vi "Log_Disdrometer_Raw_String.vi"(10 "FileFolder":path, 11 "Response":string) -> (0 "error out":errorcluster)   [LabVIEW 2018]
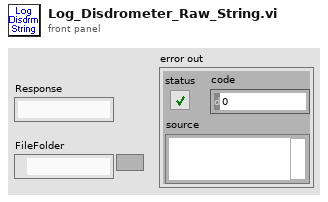
[diagram p1: front panel]
types:
  T1 = enum16{"open", "replace", "create", "open or create", "replace or create", "replace or create with confirmation"}
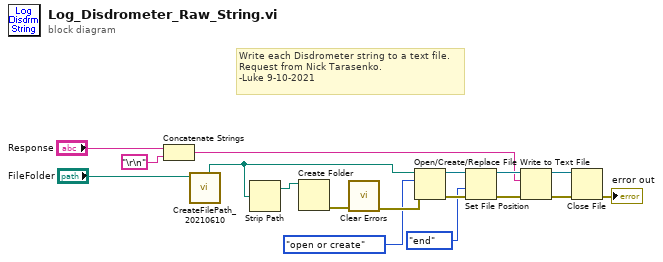
[diagram p0: block diagram]
diagram:
  # "Write each Disdrometer string to a text file.\nRequest from Nick Tarasenko. \n-Luke 9-10-2021"
  n1 = Concatenate Strings("Response", "\r\n") -> (w5:string)
  n2 = call "CreateFilePath_20210610.vi"("base path"="FileFolder") -> ("Disdrom_Raw_String_File"=w17:path)  [unwired: 6 in, 4 out]
  n3 = Strip Path(path=w17) -> (stripped path=w7:path)  [unwired: 1 out]
  n4 = Create Folder(path (use dialog)=w7) -> (error out=w8:errorcluster)  [unwired: 2 in, 2 out]
  n5 = call <vilib>:"Clear Errors.vi"("error in (no error)"=w8) -> ("error out"=w16:errorcluster)  [unwired: 5 in, 1 out]
  n6 = Open/Create/Replace File(file path (use dialog)=w17, error in=w16, operation (0:open)=T1."open or create") -> (refnum out=w9:refnum<file>, error out=w12:errorcluster)  [unwired: 3 in, 1 out]
  n7 = Set File Position(refnum=w9, from (0:start)=enum16{"start", "end", "current"}."end", error in=w12) -> (refnum out=w10:refnum<file>, error out=w13:errorcluster)  [unwired: 1 in]
  n8 = Write to Text File(file (use dialog)=w10, text=w5, error in=w13) -> (refnum out=w15:refnum<file>, error out=w14:errorcluster)  [unwired: 1 in, 1 out]
  n9 = Close File(refnum=w15, error in=w14) -> (error out=→"error out":errorcluster)  [unwired: 1 out]
